vi "Copy_Proj_Data.vi"(8 "error in (no error)":errorcluster, 9 "IB_Destination.lvclass":refnum<class "IB_Destination.lvclass">, 10 "IB_Tree_Item_Proj in":refnum<class "IB_Tree_Item_Proj.lvclass">, 11 "IB_CtrFile in":refnum<class "IB_CtrFile.lvclass">) -> (0 "error out":errorcluster, 3 "IB_CtrFile out":refnum<class "IB_CtrFile.lvclass">)   [LabVIEW 2020, in "IB_CtrFile.lvclass"]
uses:
  <vilib>/AppBuilder/IB_Classes/Source/File/CtrFile/IB_CtrFile.lvclass
  <vilib>/AppBuilder/IB_Classes/Source/File/CtrFile/IB_CtrFile.lvclass/IB_CtrFile.ctl
  <vilib>/AppBuilder/IB_Classes/Source/File/IB_Source_File.lvclass
  <vilib>/AppBuilder/IB_Classes/Source/IB_Source.lvclass
  <vilib>/AppBuilder/IB_Classes/Tree_Item_Proj_Contained_File/IB_Tree_Item_Proj_Contained_File.lvclass
  <vilib>/AppBuilder/IB_Classes/Tree_Item/IB_Tree_Item.lvclass
  e:/builds/penguin/labview/branches/2020/dev/dist/vi.lib/AppBuilder/IB_Classes/Source/File/IB_Source_File.lvclass
  e:/builds/penguin/labview/branches/2020/dev/dist/vi.lib/AppBuilder/IB_Classes/Source/IB_Source.lvclass
  e:/builds/penguin/labview/branches/2020/dev/dist/vi.lib/AppBuilder/IB_Classes/Source/File/CtrFile/IB_CtrFile.lvclass
  <vilib>/AppBuilder/IB_Classes/Tree_Item_Virtual_Folder/IB_Tree_Item_Virtual_Folder.lvclass
  e:/builds/penguin/labview/branches/2020/dev/dist/vi.lib/AppBuilder/IB_Classes/Tree_Item/IB_Tree_Item.lvclass
  e:/builds/penguin/labview/branches/2020/dev/dist/vi.lib/AppBuilder/IB_Classes/Tree_Item_Virtual_Folder/IB_Tree_Item_Virtual_Folder.lvclass
  <vilib>/AppBuilder/IB_Classes/Tree_Item_Proj/IB_Tree_Item_Proj.lvclass
  <vilib>/AppBuilder/IB_Classes/Destination/IB_Destination.lvclass
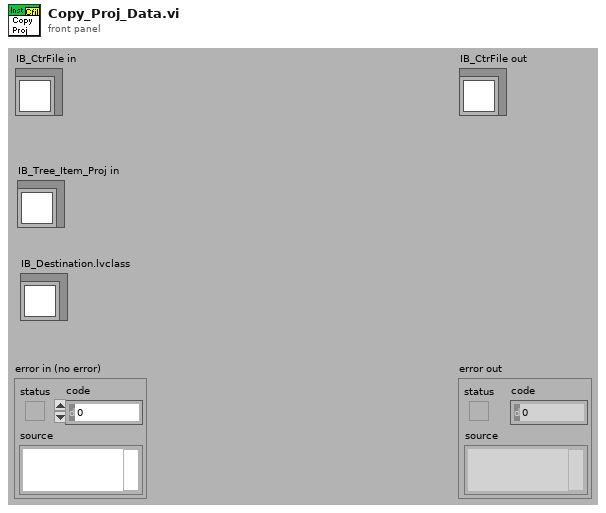
[diagram p1: front panel]
types:
  T1 = typedef "IB_Source.ctl" = cluster{"name":string, "sourceTag":string, "destTag":string, "path":path, "eng_installPath":string, "UI_inBuild?":bool, "str ref?":bool}
  T2 = typedef "IB_Tree_Item_Proj_Contained_File.ctl" = cluster{"virt folders":refnum<class "IB_Tree_Item_Virtual_Folder.lvclass">[]}
  T3 = typedef "IB_Tree_Item.ctl" = cluster{"symbol index":i32, "child tag":string, "parentTag":string, "left cell name":string}
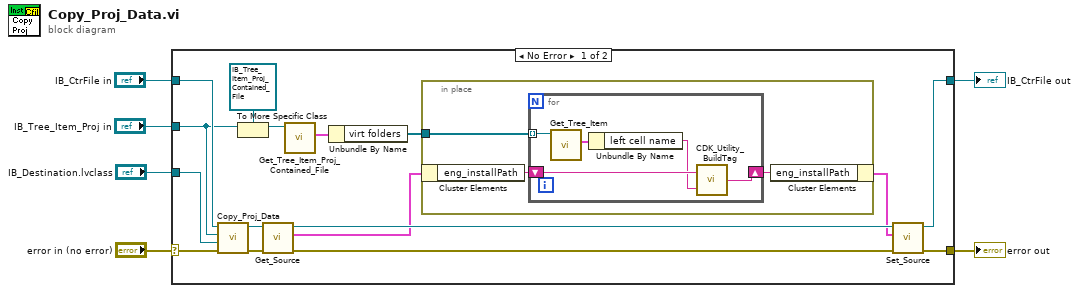
[diagram p0: block diagram]
diagram:
  n1 = case shown="No Error" "error in (no error)" {
    selector: "error in (no error)" -> [w20 w32]
    tunnel: [w12 w32] -> w6
    tunnel: [w10 w31] -> w5
    tunnel: "IB_Destination.lvclass" -> [w22 _]
    tunnel: "IB_Tree_Item_Proj in" -> [w17 _]
    tunnel: "IB_CtrFile in" -> [w21 w31]
    frame No Error {
      n2 = call-parent "Copy_Proj_Data.vi"("error in (no error)"=w20, "IB_Destination.lvclass"=w22, "IB_Tree_Item_Proj in"=w17, "IB_Source in"=w21) -> ("error out"=w19:errorcluster, "IB_Source out"=w15:refnum<class "IB_CtrFile.lvclass">)  [unwired: 6 in]
      n3 = To More Specific Class(target class=refnum<class "IB_Tree_Item_Proj_Contained_File.lvclass"> refnum ("IB_Tree_Item_Proj_Contained_File.lvclass"), reference=w17) -> (specific class reference=w16:refnum<class "IB_Tree_Item_Proj_Contained_File.lvclass">)  [unwired: 1 in, 1 out]
      n4 = call <vilib>:"Get_Source.vi"("error in (no error)"=w19, "IB_Source in"=w15) -> ("error out"=w13:errorcluster, "data"=w8:T1, "IB_Source out"=w11:refnum<class "IB_CtrFile.lvclass">)  [unwired: 7 in]
      n5 = call <vilib>:"Get_Tree_Item_Proj_Contained_File.vi"("IB_Tree_Item_Proj_Contained_File in"=w16) -> ("data"=w14:T2)  [unwired: 8 in, 2 out]
      n6 = Unbundle By Name(w14) -> ("virt folders"=w9:refnum<class "IB_Tree_Item_Virtual_Folder.lvclass">[])
      n7 = in-place {
        in-place-border: w9 -> [w25]
        n8 = in-place-cluster #1(w8) -> ("eng_installPath"=w24:string)
        n9 = for {
          tunnel: w25 -> [w30] mode=indexing
          shift-right: [w26] -> w23
          shift-left: w24 -> [w28]
          n10 = call <vilib>:"Get_Tree_Item.vi"("IB_TreeItem in"=w30) -> ("data"=w29:T3)  [unwired: 8 in, 2 out]
          n11 = Unbundle By Name(w29) -> ("left cell name"=w27:string)
          n12 = call <resource>:"CDK_Utility_BuildTag.vi"("name or relative path"=w27, "BasePath"=w28) -> ("appended path"=w26:string)
        }
        n13 = in-place-cluster #1("eng_installPath"=w23) -> (w7:T1)
      }
      n14 = call <vilib>:"Set_Source.vi"("error in (no error)"=w13, "data"=w7, "IB_Source in"=w11) -> ("error out"=w12:errorcluster, "IB_Source out"=w10:refnum<class "IB_CtrFile.lvclass">)  [unwired: 7 in]
    }
    frame Error {
    }
  }
  "error out" <- w6
  "IB_CtrFile out" <- w5
